vi "data without drive coil times.vi"(6 "buffer (us) before":dbl=-20000.0 format="%#_13g", 7 "buffer (us) after":dbl=100000.0 format="%#_13g", 8 "error in (no error)":errorcluster, 10 "coil":T1, 11 "data":T1) -> (0 "error out":errorcluster, 2 "not currently in coil veto":bool, 3 "data_no_coil":T2[](array[typedef]))   [LabVIEW 2017]
uses:
  typedefs/reading.ctl
  typedefs/readingType.ctl
  typedefs/reading queue.ctl
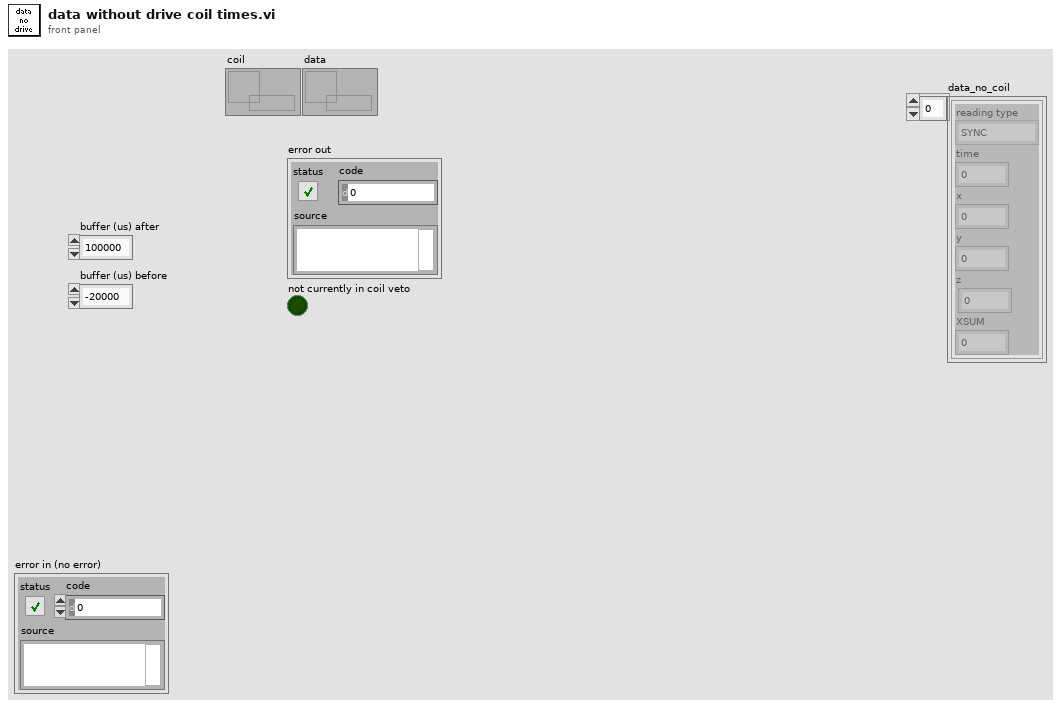
[diagram p1: front panel]
types:
  T1 = typedef "reading queue.ctl" = refnum<queue>
  T2 = typedef "reading.ctl" = cluster{"reading type":T3, "time":fxp<+,48,48>, "x":sgl, "y":sgl, "z":sgl, "XSUM":u8}
  T3 = typedef "readingType.ctl" = enum8{"SYNC", "DETVAL", "COILI", "MAGVEC", "ACCVEC"}
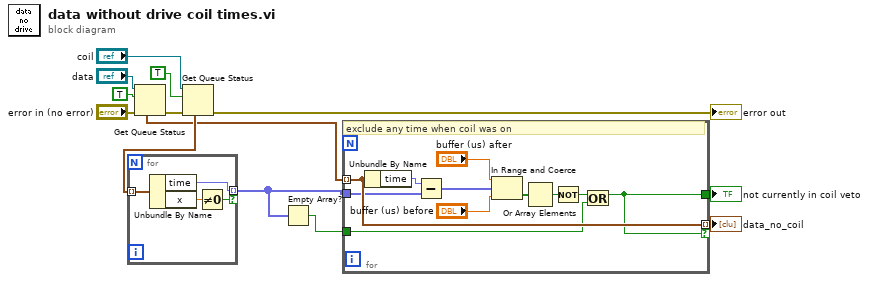
[diagram p0: block diagram]
diagram:
  n1 = Get Queue Status(queue="data", return elements? (F)=TRUE, error in (no error)="error in (no error)") -> (error out=w11:errorcluster, elements=w5:T2[])  [unwired: 6 out]
  n2 = Get Queue Status(queue="coil", return elements? (F)=TRUE, error in (no error)=w11) -> (error out=→"error out":errorcluster, elements=w9:T2[])  [unwired: 6 out]
  n3 = for {
    tunnel: w9 -> [w16] mode=indexing
    tunnel: [w14] -> w2 mode=indexing if=w15
    n4 = Unbundle By Name(w16) -> ("time"=w14:fxp<+,48,48>, "x"=w17:sgl)
    n5 = Not Equal To 0?(x=w17) -> (x != 0?=w15:bool)
  }
  n6 = Empty Array?(array=w2) -> (empty?=w1:bool)
  n7 = for {
    tunnel: w5 -> [w28] mode=indexing
    tunnel: [w28] -> w6 mode=indexing if=w19
    tunnel: w2 -> [w26]
    tunnel: [w19] -> w7
    tunnel: w1 -> [w18]
    # "exclude any time when coil was on"
    n8 = Unbundle By Name(w28) -> ("time"=w27:fxp<+,48,48>)
    n9 = Subtract(x=w27, y=w26) -> (x-y=w25:fxp<+/-,49,49>[])
    n10 = In Range and Coerce(upper limit="buffer (us) after", x=w25, lower limit="buffer (us) before") -> (In Range?=w22:bool[])  [unwired: 1 out]
    n11 = Or Array Elements(Boolean array=w22) -> (logical OR=w21:bool)
    n12 = Not(x=w21) -> (.not. x?=w20:bool)
    n13 = Or(x=w20, y=w18) -> (x .or. y?=w19:bool)
  }
  "data_no_coil" <- w6
  "not currently in coil veto" <- w7
